vi "arduino.vi"() -> ()   [LabVIEW 2017]
uses:
  <vilib>/Instr/_visa.llb/VISA Flush IO Buffer Mask.ctl
  <vilib>/Utility/error.llb/DialogType.ctl
  <vilib>/Instr/_visa.llb/VISA Configure Serial Port (Instr).vi
panel:
  out "Thermometer":dbl[unit](slide) scale=0.0..100.0
  out "temp":dbl[unit](slide) scale=0.0..100.0
  out "light":dbl(knob) caption="x+y" scale=0.0..1000.0
  out "input array":u8[][](array[numeric])
  out "Serial Settings:Number of Bytes at Serial Port":u32(graph)
  out "Numeric":u8
  in  "Ring":u16(ring) items=["Pot", "Button"]
  in  "Array":bool[][](array[boolean])
  out "number":dbl(knob) scale=0.0..1000.0
  out "Waveform Chart":dbl(graph)
  out "Data  String":string
  in  "VISA resource name":refnum<visa-resource-name>
  in  "stop":bool
  # "potentiometer"
  # "light sensor"
  # "temperature sensor"
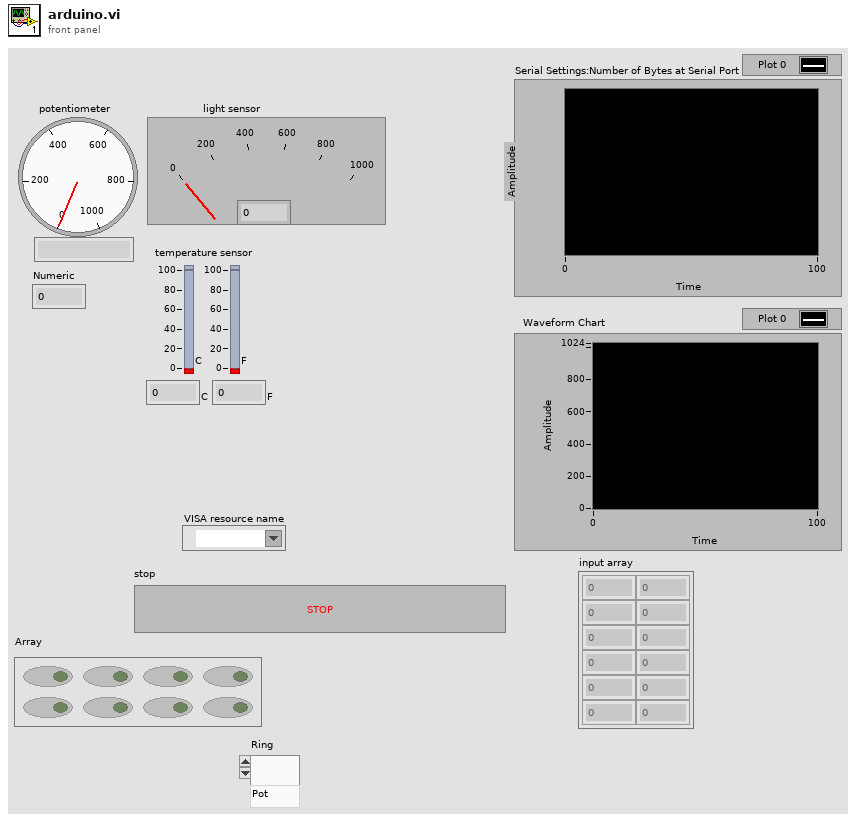
[diagram p1: front panel]
types:
  T1 = typedef "DialogType.ctl" = u16
  T2 = typedef "VISA Flush IO Buffer Mask.ctl" = u16
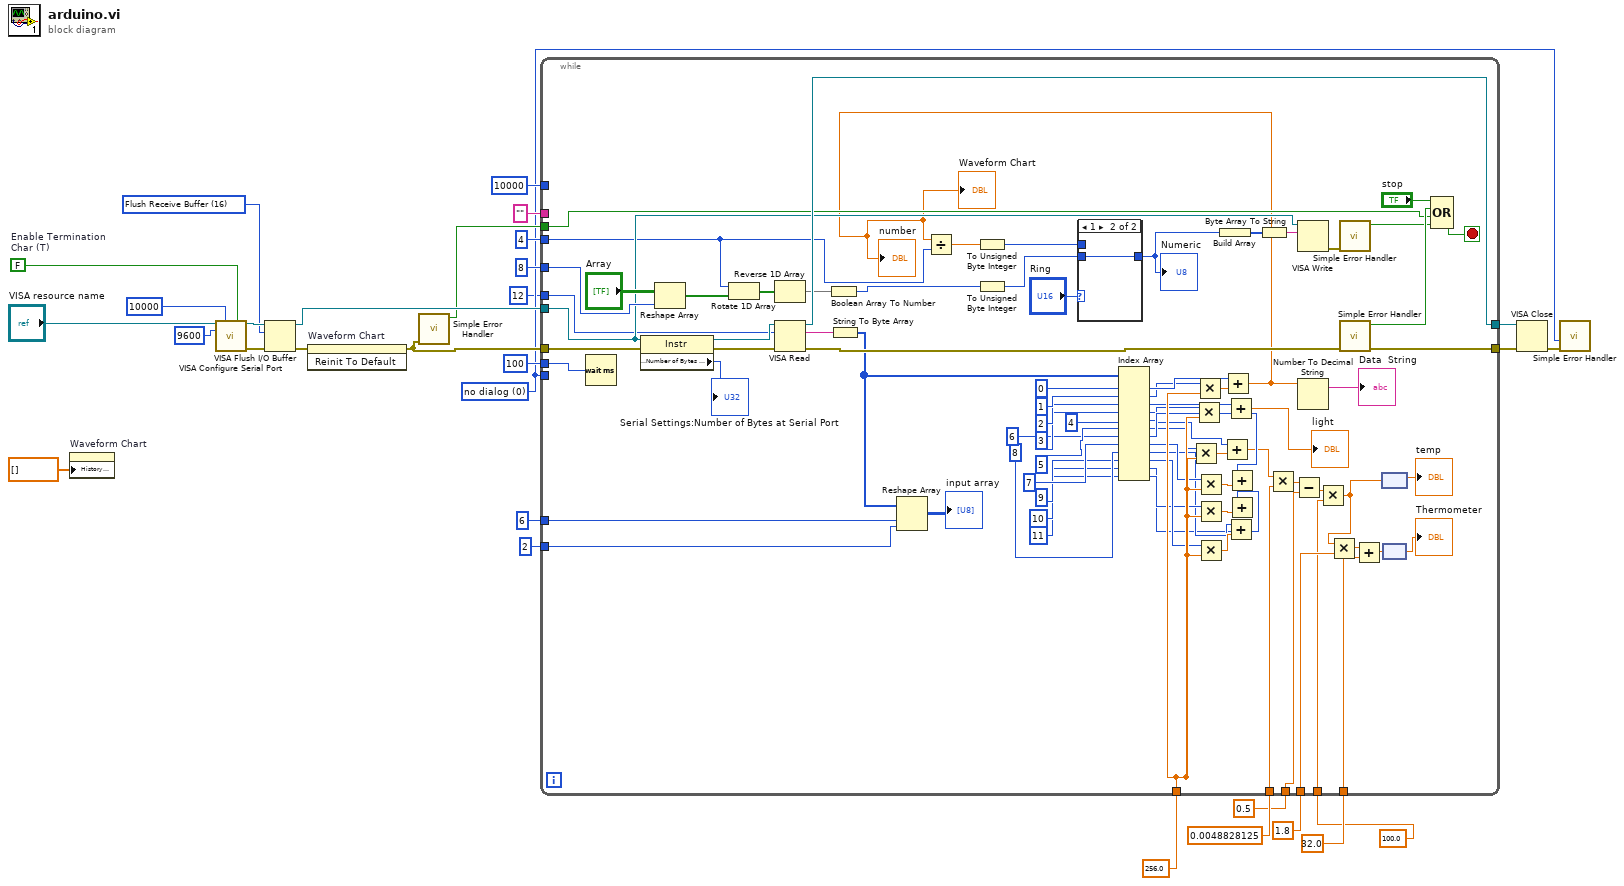
[diagram p0: block diagram]
diagram:
  w9 = FALSE  # Enable Termination Char (T)
  w12 = T1 0 items=["no dialog", "OK message", "continue or stop message", "OK message + warnings", "continue/stop + warnings"] ("type of dialog (OK msg:1)")
  w20 = T2 16 items=["Flush Receive Buffer"=16, "Write Transmit Buffer to Device"=32, "Flush Receive Buffer (No I/O)"=64, "Flush Transmit Buffer"=128] ("Mask")
  n1 = property on="Waveform Chart" class="WFChart (strict)"("History Data"=dbl[] []) -> ()  [unwired: 2 in, 2 out]
  n2 = call-poly "VISA Configure Serial Port"("VISA resource name"="VISA resource name", "timeout (10sec)"=u32 10000, "Enable Termination\nChar (T)"=w9, "baud rate (9600)"=9600) -> ("VISA resource name out"=w21:refnum<visa-resource-name>, "error out"=w22:errorcluster)  [unwired: 10 in]
  n3 = VISA Flush I/O Buffer(VISA resource name=w21, mask (16)=w20, error in (no error)=w22) -> (VISA resource name out=w19:refnum<visa-resource-name>, error out=w16:errorcluster)
  n4 = invoke on="Waveform Chart" class="WFChart (strict)" method="Reinit To Default"(error in=w16) -> (error out=w14:errorcluster)  [unwired: 2 in, 2 out]
  n5 = call <vilib>:"Simple Error Handler.vi"("error in (no error)"=w14) -> ("error?"=w13:bool)  [unwired: 4 in, 4 out]
  n6 = while {
    tunnel: w19 -> [w92]
    tunnel: "" ("string") -> [_]
    tunnel: [w90] -> w26
    tunnel: [w111] -> w25
    tunnel: u8 4 ("x") -> [w82]
    tunnel: 100 -> [w110]
    tunnel: w14 -> [w106]
    tunnel: u32 10000 ("timeout (0)") -> [_]
    tunnel: 8 -> [w97]
    tunnel: w13 -> [w85]
    tunnel: w12 -> [_]
    tunnel: 12 -> [w88]
    tunnel: 6 ("dimension size") -> [w80]
    tunnel: 2 ("dimension size") -> [w81]
    tunnel: 256.0 ("y") -> [w65]
    tunnel: 32.0 ("y") -> [w43]
    tunnel: 1.8 ("y") -> [w42]
    tunnel: 0.0048828125 ("y") -> [w38]
    tunnel: 100.0 ("y") -> [w32]
    tunnel: 0.5 ("y") -> [w31]
    stop <- w91 stop-if-true
    n7 = Wait (ms)(milliseconds to wait=w110) -> ()  [unwired: 1 out]
    n8 = property class="Instr"(reference=w92, error in=w106) -> (reference out=w108:refnum<visa-resource-name>, error out=w107:errorcluster, "Serial Settings:Number of Bytes at Serial Port"=→"Serial Settings:Number of Bytes at Serial Port":u32)
    n9 = Reshape Array("Array", w97) -> (w99:bool[])
    n10 = Rotate 1D Array(1:w99, 2:w82) -> (0:w96:bool[])
    n11 = Reverse 1D Array(array=w96) -> (reversed array=w95:bool[])
    n12 = VISA Read(VISA resource name=w108, byte count=w88, error in (no error)=w107) -> (VISA resource name out=w111:refnum<visa-resource-name>, read buffer=w87:string, error out=w89:errorcluster)  [unwired: 1 out]
    n13 = Boolean Array To Number(Boolean array=w95) -> (number=w101:u32)
    n14 = String To Byte Array(string=w87) -> (unsigned byte array=w78:u8[])
    n15 = Reshape Array(w78, w80, w81) -> (→"input array":u8[][])
    n16 = To Unsigned Byte Integer(number=w101) -> (unsigned 8bit integer=w100:u8)
    n17 = Index Array(array=w78, index #1=0 ("index"), index #2=1 ("index"), index #3=2 ("index"), index #4=3 ("index"), index #5=4 ("index"), index #6=5 ("index"), index #7=6 ("index"), index #8=7 ("index"), index #9=8 ("index"), index #10=9 ("index"), index #11=10 ("index"), index #12=11 ("index")) -> (element #1=w50:u8, element #2=w49:u8, element #3=w57:u8, element #4=w48:u8, element #5=w36:u8, element #6=w37:u8, element #7=w56:u8, element #8=w64:u8, element #9=w55:u8, element #10=w63:u8, element #11=w54:u8, element #12=w62:u8)
    n18 = Multiply(x=w37, y=w65) -> (x*y=w58:dbl)
    n19 = Multiply(x=w48, y=w65) -> (x*y=w52:dbl)
    n20 = Multiply(x=w49, y=w65) -> (x*y=w51:dbl)
    n21 = Multiply(x=w64, y=w65) -> (x*y=w59:dbl)
    n22 = Multiply(x=w62, y=w65) -> (x*y=w61:dbl)
    n23 = Multiply(x=w63, y=w65) -> (x*y=w60:dbl)
    n24 = Add(x=w36, y=w58) -> (x+y=w39:dbl)
    n25 = Add(x=w50, y=w51) -> (x+y=w47:dbl)
    "Waveform Chart" <- w47
    "number" <- w47
    n26 = Divide(x=w47, y=w82) -> (x/y=w102:dbl)
    n27 = To Unsigned Byte Integer(number=w102) -> (unsigned 8bit integer=w104:u8)
    n28 = case shown="1" "Ring" {
      tunnel: [w113 w114] -> w103
      tunnel: w104 -> [w113 _]
      tunnel: w100 -> [_ w114]
      frame 0, Default {
      }
      frame 1 {
      }
    }
    "Numeric" <- w103
    n29 = Build Array(w103) -> (w93:u8[])
    n30 = Add(x=w57, y=w52) -> (x+y=→"light":dbl)
    n31 = Add(x=w55, y=w60) -> ()  [unwired: 1 out]
    n32 = Add(x=w56, y=w59) -> ()  [unwired: 1 out]
    n33 = Add(x=w54, y=w61) -> ()  [unwired: 1 out]
    n34 = Byte Array To String(unsigned byte array=w93) -> (string=w105:string)
    n35 = Multiply(x=w39, y=w38) -> (x*y=w35:dbl)
    n36 = Subtract(x=w35, y=w31) -> (x-y=w34:dbl)
    n37 = VISA Write(VISA resource name=w92, write buffer=w105) -> (error out=w84:errorcluster)  [unwired: 1 in, 2 out]
    n38 = Number To Decimal String(number=w47) -> (decimal integer string=→"Data  String":string)  [unwired: 1 in]
    n39 = Multiply(x=w34, y=w32) -> (x*y=w33:dbl)
    n40 = Multiply(x=w33, y=w42) -> (x*y=w44:dbl)
    n41 = call <vilib>:"Simple Error Handler.vi"("error in (no error)"=w84) -> ("error?"=w83:bool)  [unwired: 4 in, 4 out]
    n42 = call <vilib>:"Simple Error Handler.vi"("error in (no error)"=w89) -> ("error?"=w86:bool, "error out"=w90:errorcluster)  [unwired: 4 in, 3 out]
    n43 = Add(x=w44, y=w43) -> (x+y=w41:dbl)
    n44 = node(w33) -> (→"temp":dbl[unit])
    n45 = node(w41) -> (→"Thermometer":dbl[unit])
    n46 = Compound Arithmetic op=OR("stop", w86, w85, w83) -> (w91:bool)
  }
  n47 = VISA Close(VISA resource name=w25, error in (no error)=w26) -> (error out=w27:errorcluster)
  n48 = call <vilib>:"Simple Error Handler.vi"("type of dialog (OK msg:1)"=w12, "error in (no error)"=w27) -> ()  [unwired: 3 in, 5 out]
